vi "DETStatus-Com-Exec.vi"(8 "error in (no error)":errorcluster, 11 "DAQmxTaskContainer in":refnum<class "DAQmxTaskContainer.lvclass">) -> (0 "error out":errorcluster, 3 "DAQmxTaskContainer out":refnum<class "DAQmxTaskContainer.lvclass">)   [LabVIEW 2015, in "DAQmxTaskContainer.lvclass"]
uses:
  DAQmxTaskContainer.lvclass
  dependecies/ControlsVIs/Clusters-def/DAQmx-Reply-Connect-client.ctl
  dependecies/ControlsVIs/Clusters-def/SERVER-Commands.ctl
  dependecies/ControlsVIs/Clusters-def/Message types.ctl
  DAQmxTask.lvclass
  Message/Message.lvclass
  Control/Control-Server/Control-Server.lvclass
  GeneralFunctionality/GeneralFunctionality.lvclass
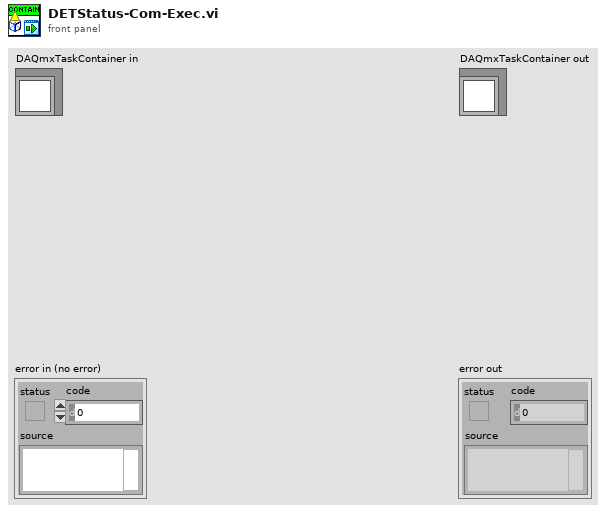
[diagram p1: front panel]
types:
  T1 = typedef "Message types.ctl" = string
  T2 = typedef "Control-Server.lvclass/SERVER-Commands.ctl" = string
  T3 = typedef "DAQmxTaskContainer.lvclass/DAQmx-Reply-Connect-client.ctl" = cluster{"on/off":bool, "RelayKeyHeater/off":bool, "LaserShutter":bool, "AcceleratorShutter":bool, "Power":bool, "Faraday Cup Status":bool, "error":errorcluster}
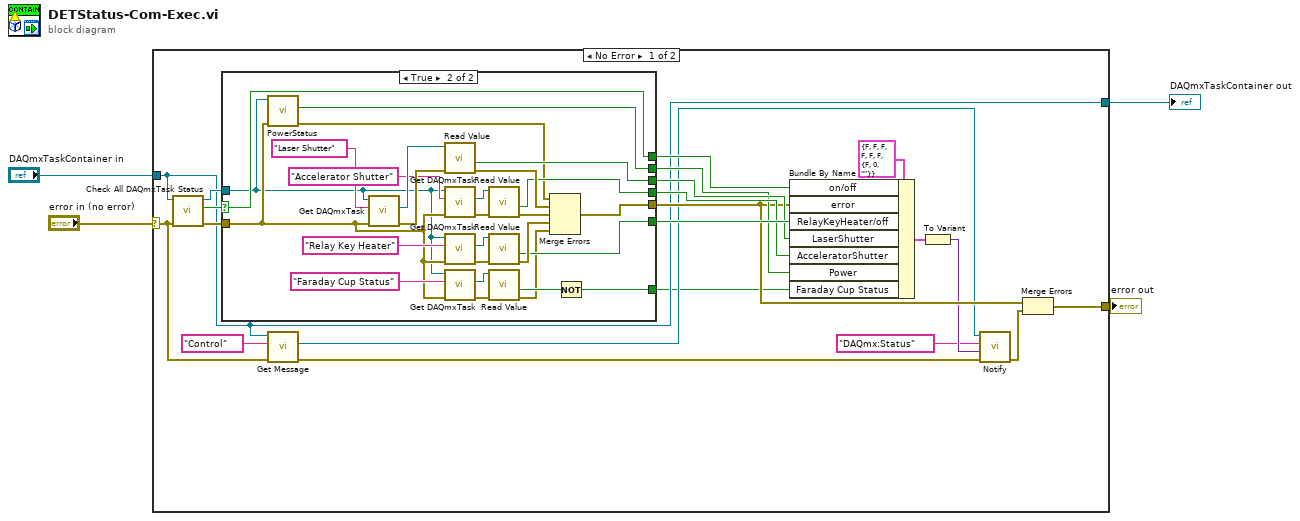
[diagram p0: block diagram]
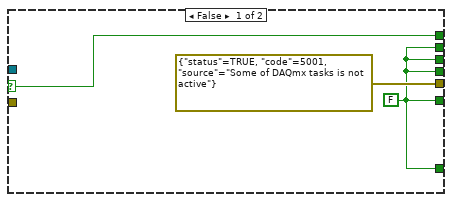
[diagram p2: hidden frame]
diagram:
  n1 = case shown="No Error" "error in (no error)" {
    selector: "error in (no error)" -> [w14 w57]
    tunnel: [w7 w57] -> w3
    tunnel: [w13 w56] -> w1
    tunnel: "DAQmxTaskContainer in" -> [w13 w56]
    frame No Error {
      n2 = call "Check All DAQmxTask Status.vi"("error in (no error)"=w14, "DAQmxTaskContainer en entrée"=w13) -> ("error out"=w20:errorcluster, "All active"=w19:bool, "DAQmxTaskContainer en sortie"=w18:refnum<class "DAQmxTaskContainer.lvclass">)  [unwired: 6 in, 1 out]
      n3 = case shown="True" w19 {
        selector: w19 -> [w27 w37]
        tunnel: [errorcluster {"status"=TRUE, "code"=5001, "source"="Some of DAQmx tasks is not active"} ("error IO") w43] -> w16
        tunnel: [w26 w38] -> w21
        tunnel: [w26 w42] -> w22
        tunnel: [w26 w41] -> w23
        tunnel: [w26 w40] -> w24
        tunnel: w20 -> [_ w34]
        tunnel: w18 -> [_ w30]
        tunnel: [w27 w37] -> w17
        tunnel: [w26 w29] -> w5
        frame False {
          w26 = FALSE ("Data")
        }
        frame True {
          n4 = call "PowerStatus.vi"("error in (no error)"=w34, "DAQmxTaskContainer in"=w30) -> ("error out"=w39:errorcluster, "On/Off"=w38:bool)  [unwired: 7 in, 1 out]
          n5 = call "Get DAQmxTask.vi"("error in (no error)"=w34, "Task name"="Laser Shutter", "DAQmxTaskContainer in"=w30) -> ("error out"=w47:errorcluster, "DAQmx Task"=w48:refnum<class "DAQmxTask.lvclass">)  [unwired: 6 in, 1 out]
          n6 = call-dynamic "Read Value.vi"("error in (no error)"=w47, "DAQmxTask en entrée"=w48) -> ("error out"=w53:errorcluster, "Data"=w42:bool)  [unwired: 6 in, 2 out]
          n7 = call "Get DAQmxTask.vi"("error in (no error)"=w34, "Task name"="Accelerator Shutter", "DAQmxTaskContainer in"=w30) -> ("error out"=w49:errorcluster, "DAQmx Task"=w50:refnum<class "DAQmxTask.lvclass">)  [unwired: 6 in, 1 out]
          n8 = call "Get DAQmxTask.vi"("error in (no error)"=w34, "Task name"="Relay Key Heater", "DAQmxTaskContainer in"=w30) -> ("error out"=w51:errorcluster, "DAQmx Task"=w52:refnum<class "DAQmxTask.lvclass">)  [unwired: 6 in, 1 out]
          n9 = call "Get DAQmxTask.vi"("error in (no error)"=w34, "Task name"="Faraday Cup Status", "DAQmxTaskContainer in"=w30) -> ("error out"=w32:errorcluster, "DAQmx Task"=w36:refnum<class "DAQmxTask.lvclass">)  [unwired: 6 in, 1 out]
          n10 = call-dynamic "Read Value.vi"("error in (no error)"=w49, "DAQmxTask en entrée"=w50) -> ("error out"=w54:errorcluster, "Data"=w41:bool)  [unwired: 6 in, 2 out]
          n11 = call-dynamic "Read Value.vi"("error in (no error)"=w51, "DAQmxTask en entrée"=w52) -> ("error out"=w55:errorcluster, "Data"=w40:bool)  [unwired: 6 in, 2 out]
          n12 = call-dynamic "Read Value.vi"("error in (no error)"=w32, "DAQmxTask en entrée"=w36) -> ("error out"=w31:errorcluster, "Data"=w33:bool)  [unwired: 6 in, 2 out]
          n13 = Merge Errors(w39, w53, w54, w55, w31) -> (w43:errorcluster)
          n14 = Not(x=w33) -> (.not. x?=w29:bool)
        }
      }
      n15 = call "Get Message.vi"("error in (no error)"=w14, "Message type"=T1 "Control", "GeneralFunctionality en entrée"=w13) -> ("error out"=w11:errorcluster, "Message.lvclass"=w12:refnum<class "Message.lvclass">)  [unwired: 6 in, 1 out]
      n16 = Bundle By Name(cluster=T3 {"on/off"=FALSE, "RelayKeyHeater/off"=FALSE, "LaserShutter"=FALSE, "AcceleratorShutter"=FALSE, "Power"=FALSE, "Faraday Cup Status"=FALSE, "error"={"status"=FALSE, "code"=0, "source"=""}} ("output cluster"), "on/off"=w17, "error"=w16, "RelayKeyHeater/off"=w24, "LaserShutter"=w22, "AcceleratorShutter"=w23, "Power"=w21, "Faraday Cup Status"=w5) -> (w15:T3)
      n17 = To Variant(anything=w15) -> (Variant=w10:variant)
      n18 = call "Notify.vi"("error in (no error)"=w11, "Data"=w10, "command"=T2 "DAQmx:Status" ("Commands"), "Message en entrée"=w12) -> ("error out"=w8:errorcluster)  [unwired: 6 in, 1 out]
      n19 = Merge Errors(w16, w8) -> (w7:errorcluster)
    }
    frame Error {
    }
  }
  "error out" <- w3
  "DAQmxTaskContainer out" <- w1
